vi "Laser_COM.vi"() -> ()   [LabVIEW 2014]
uses:
  <vilib>/Instr/_visa.llb/Select Event Type.ctl
  <vilib>/Instr/_visa.llb/VISA Configure Serial Port (Instr).vi
panel:
  out "7":bool
  out "6":bool
  out "4":bool
  out "5":bool
  out "3":bool
  out "2":bool
  out "1":bool
  out "0":bool
  in  "Control PL":bool
  out "DB25 PL":bool
  out "RS232 PL":bool
  out "DB25 GL":bool
  out "RS232 GL":bool
  in  "Control GL":bool
  out "DB25 ML":bool
  out "RS232 ML":bool
  in  "Control ML":bool
  out "on/off? 5":bool
  in  "Laser":bool
  out "Laser EM":bool caption="Излучение включено!"
  out "on/off? 3":bool
  out "on/off? 2":bool
  in  "Send":bool
  in  "write buffer":string caption="Передать команду"
  out "COM_connect":bool
  in  "Connect":bool
  out "SN:":string
  out "ID:":string
  out "Guide  laser":bool
  out "module temp":dbl caption="Темп. модуля" format="%#_g °C"
  in  "Power":dbl(slide) caption="Мощность излучения, %" min=0.0 max=100.0 step=0.5 scale=0.0..100.0 scale format="%#.2g"
  in  "Laser pilot":bool caption="Лазер пилот"
  in  "COM":refnum<visa-resource-name>="COM1" caption="Laser COM-port"
  out "read buffer":string caption="ОТВЕТ:"
  out "error out":errorcluster
  in  "error in (no error)":errorcluster
  # "ID:\n\nSN:"
  # "Блок  управления основным лазером"
  # "RS-232"
  # "DB-25"
  # "T модуля -"
  # "RS-232"
  # "Мощьность  излучения, %"
  # "DB-25"
  # "DB-25"
  # "Пилот Лазер"
  # "RS-232"
  # "DB-25"
  # "Терминал"
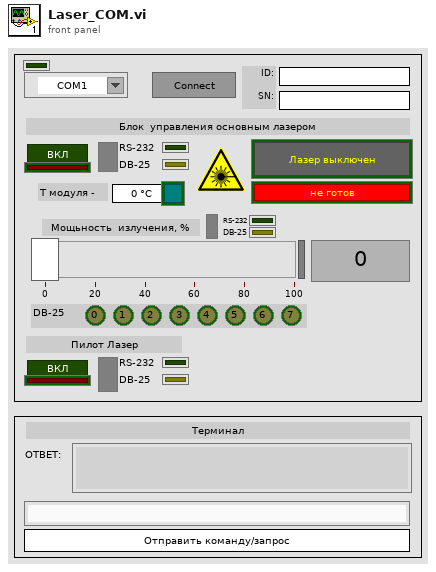
[diagram p1: front panel]
types:
  T1 = typedef "Select Event Type.ctl" = u32
  T2 = cluster{"Power control by DB-25":bool, "Reserved[1]":bool, "AuxOFF control by DB-25":bool, "Guide laser control by DB-25":bool, "Reserved[4]":bool, "Reserved[5]":bool, "Reserved[6]":bool, "Emission Modulation control by DB-25":bool, "The laser is in Jump PRR mode":bool, "Reserved[9]":bool, "Bitstream 1 (BS1) mode is active":bool, "Reserved[11]":bool, "PRR controlled by Sync line in DB-25":bool, "Emission Enable control by DB-25":bool, "APD mode is controlled by DB-25":bool, "Automatic latch":bool, "Reserved[16]":bool, "Reserved[17]":bool, "Reserved[18]":bool, "The laser is in Sweep PRR mode":bool, "The laser is in Follow PRR mode":bool, "Manual Prepump mode is active":bool, "Manual residual is controlled by DB-25":bool, "Reserved[23]":bool, "Reserved[24]":bool, "Guide laser safety function is not activated":bool, "Discharge circuit safety function is activated":bool, "Reserved[27]":bool, "Reserved[28]":bool, "Reserved[29]":bool, "Reserved[30]":bool, "Reserved[31]":bool}
  T3 = cluster{"Rack  reflection":bool, "Temp Laser module":bool, "Temp Laser head":bool, "System Alarm":bool, "+24V main supply Alarm":bool, "HK supply  Alarm":bool, "Laser ready":bool, "Warning is activated":bool}
  T4 = cluster{"Emergency stop":bool, "External PRR [1]":bool, "External PRR [2]":bool, "Reserved [3]":bool, "Reserved [4]":bool, "Guide laser":bool, "Reserved [6]":bool, "Reserved [7]":bool, "Laser emission":bool, "Reserved [9]":bool, "Reserved [10]":bool, "Laser emission command was received by RS-232":bool, "Guide laser command was received by RS-232":bool, "24V Main supply voltage is in specified range":bool, "HK supply voltage is in specified range":bool, "Emission Enable is switched by RS-232":bool, "Reserved [16]":bool, "Reserved [17]":bool, "Reserved [18]":bool, "Reserved [19]":bool, "Reserved [20]":bool, "Reserved [21]":bool, "Reserved [22]":bool, "Reserved [23]":bool, "Reserved [24]":bool, "Reserved [25]":bool, "Reserved [26]":bool, "Reserved [27]":bool, "Reserved [28]":bool, "Reserved [29]":bool, "Reserved [30]":bool, "Reserved [31]":bool}
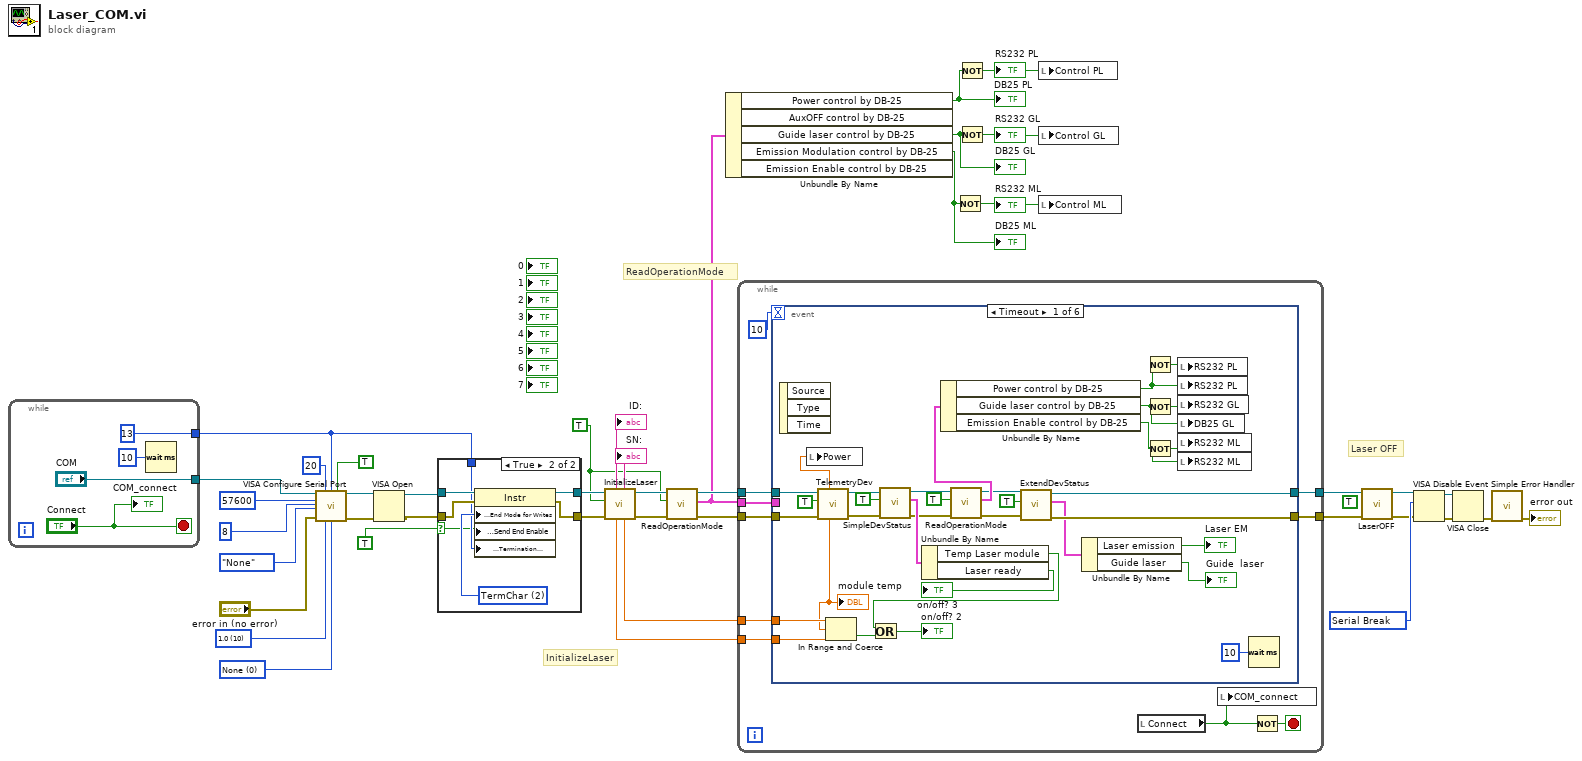
[diagram p0: block diagram]
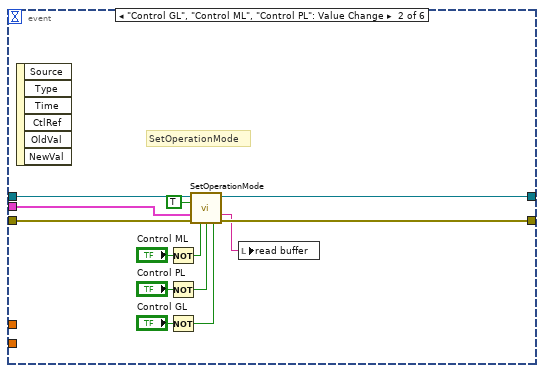
[diagram p2: hidden frame]
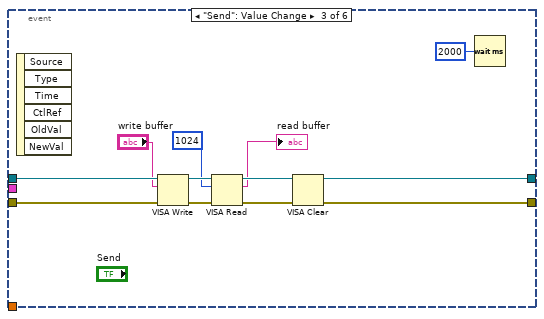
[diagram p3: hidden frame]
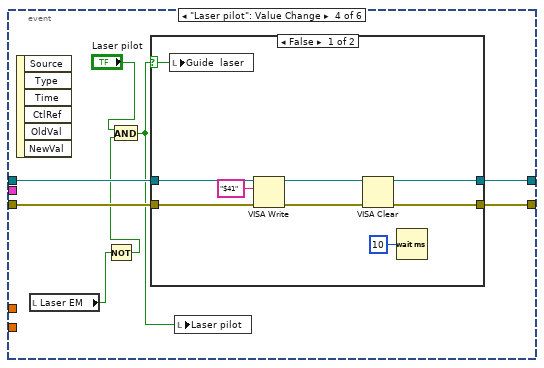
[diagram p4: hidden frame]
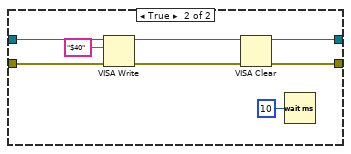
[diagram p5: hidden frame]
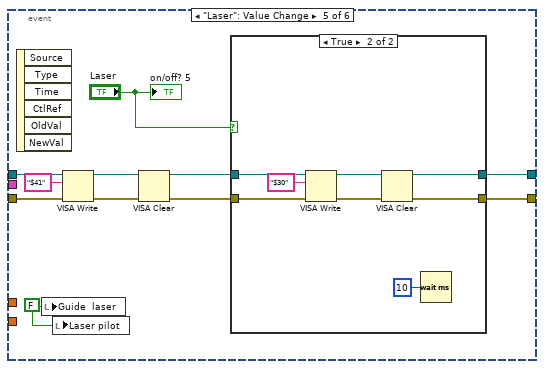
[diagram p6: hidden frame]
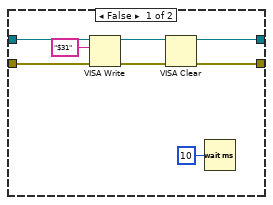
[diagram p7: hidden frame]
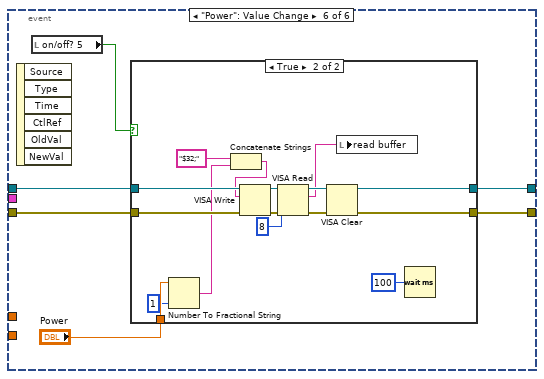
[diagram p8: hidden frame]
diagram:
  w23 = T1 1073684515 items=["Service Request"=1073684491, "Trigger"=3221168138, "Clear"=1073684493, "VXI Signal"=1073684512, "VXI/VME Interrupt"=3221168161, "VXI/VME Sysfail"=1073684509, "VXI/VME Sysreset"=1073684510, "GPIB CIC"=1073684498, "GPIB Talk"=1073684499, "GPIB Listen"=1073684500, "PXI Interrupt"=1073684514, "Serial Break"=1073684515, "Serial TermChar"=1073684516, "Serial CTS"=1073684521, "Serial DSR"=1073684522, "Serial DCD"=1073684524, "Serial RI"=1073684526, "Serial Character"=1073684533, "USB Interrupt"=1073684535, "All Enabled"=1073709055] ("Event Type")
  (unwired) TRUE
  w28 = u16 0 items=["None", "XON/XOFF", "RTS/CTS", "XON/XOFF & RTS/CTS", "DTR/DSR", "XON/XOFF & DTR/DSR"] ("flow control (0:none)")
  w10 = TRUE
  w35 = u16 10 items=["1.0"=10, "1.5"=15, "2.0"=20] ("stop bits (10: 1 bit)")
  # "Laser OFF"
  # "ReadOperationMode"
  # "InitializeLaser"
  n1 = while {
    tunnel: ["COM"] -> w27
    tunnel: [i16 13 ("term_char")] -> w26
    stop <- "Connect" stop-if-true
    n2 = Wait (ms)(milliseconds to wait=u32 10) -> ()  [unwired: 1 out]
    "COM_connect" <- "Connect"
  }
  n3 = call-poly "VISA Configure Serial Port"("VISA resource name"=w27, "timeout (10sec)"=u32 20, "termination char\n(0xA = '\\n' = LF)"=w26, "Enable Termination\nChar (T)"=TRUE ("Enable Termination\nChar (T)"), "baud rate (9600)"=u32 57600 ("baud rate"), "data bits (8)"=u16 8, "parity (0:none)"=enum16{"None", "Odd", "Even", "Mark", "Space"}."None", "error in (no error)"="error in (no error)", "stop bits (10: 1 bit)"=w35, "flow control (0:none)"=w28) -> ("VISA resource name out"=w38:refnum<visa-resource-name>, "error out"=w37:errorcluster)  [unwired: 4 in]
  n4 = VISA Open(error in (no error)=w37, VISA resource name=w38) -> (VISA resource name=w32:refnum<visa-resource-name>, error out=w33:errorcluster)  [unwired: 3 in]
  n5 = case shown="True" TRUE ("End write with termination character?") {
    selector: TRUE ("End write with termination character?") -> [_ w49]
    tunnel: w32 -> [w47 w55]
    tunnel: w33 -> [w48 w54]
    tunnel: [w47 w53] -> w21
    tunnel: [w48 w52] -> w22
    tunnel: w26 -> [_ w50]
    frame False {
    }
    frame True {
      w51 = u16 2 items=["None", "LastBit", "TermChar", "Break"] ("Serial Settings:Serial End Mode for Writes")
      n6 = property class="Instr"(reference=w55, error in=w54, "Serial Settings:End Mode for Writes"=w51, "Message Based Settings:Send End Enable"=w49, "Message Based Settings:Termination Character"=w50) -> (reference out=w53:refnum<visa-resource-name>, error out=w52:errorcluster)
    }
  }
  n7 = call "InitializeLaser.vi"("error in"=w22, "ON/OFF"=w10, "VISA resource name in"=w21) -> ("error out"=w11:errorcluster, "VISA resource name out"=w12:refnum<visa-resource-name>, "Tmax"=w20:dbl, "SN:"=→"SN:":string, "Tmin"=w19:dbl, "Лазер: ID:"=→"ID:":string)  [unwired: 1 in, 2 out]
  n8 = call "ReadOperationMode.vi"("error in"=w11, "ON/OFF"=w10, "VISA resource name in"=w12) -> ("error out"=w13:errorcluster, "Operation Mode Status"=w3:T2, "VISA resource name out"=w14:refnum<visa-resource-name>)  [unwired: 5 in, 1 out]
  n9 = Unbundle By Name(w3) -> ("Power control by DB-25"=w9:bool, "Guide laser control by DB-25"=w7:bool, "Emission Modulation control by DB-25"=w4:bool)  [unwired: 2 out]
  "DB25 GL" <- w7
  "DB25 PL" <- w9
  "DB25 ML" <- w4
  n10 = while {
    tunnel: w13 -> [w60]
    tunnel: w14 -> [w61]
    tunnel: [w63] -> w16
    tunnel: [w62] -> w15
    tunnel: w20 -> [w58]
    tunnel: w19 -> [w57]
    tunnel: w3 -> [w56]
    stop <- w65 stop-if-true
    n11 = event shown="[0] Timeout" {
      selector: _ -> [_ _ _ _ _ _]
      dyn-events: _ -> [_ _ _ _ _ _]
      timeout: 10 -> [_ _ _ _ _ _]
      tunnel: w61 -> [w74 w112 w124 w132 w159 w181]
      tunnel: w60 -> [w73 w111 w123 w131 w158 w180]
      tunnel: [w78 w109 w118 w130 w154 w179] -> w63
      tunnel: [w77 w110 w117 w129 w153 w178] -> w62
      tunnel: w57 -> [w97 _ _ _ _ _]
      tunnel: w58 -> [w98 _ _ _ _ _]
      tunnel: w56 -> [_ w106 _ _ _ _]
      event Timeout {
        n12 = event-data() -> ()  [unwired: 1 in, 3 out]
        n13 = call "TelemetryDev.vi"("error in"=w73, "ON/OFF"=TRUE, "VISA resource name in"=w74) -> ("error out"=w70:errorcluster, "VISA resource name out"=w71:refnum<visa-resource-name>, "module temp"=w69:dbl, "Laser Power,%"=w68:dbl)  [unwired: 4 in, 1 out]
        "module temp" <- w69
        n14 = local write "Power"(w68) -> ()
        n15 = In Range and Coerce(upper limit=w98, x=w69, lower limit=w97) -> (In Range?=w81:bool)  [unwired: 1 out]
        n16 = call "SimpleDevStatus.vi"("error in"=w70, "ON/OFF"=TRUE ("Boolean"), "VISA resource name in"=w71) -> ("error out"=w90:errorcluster, "Device Status"=w93:T3, "VISA resource name out"=w91:refnum<visa-resource-name>)  [unwired: 5 in]
        n17 = Unbundle By Name(w93) -> ("Temp Laser module"=w95:bool, "Laser ready"=→"on/off? 3":bool)
        n18 = Or(x=w95, y=w81) -> (x .or. y?=→"on/off? 2":bool)
        n19 = call "ReadOperationMode.vi"("error in"=w90, "ON/OFF"=TRUE, "VISA resource name in"=w91) -> ("error out"=w79:errorcluster, "Operation Mode Status"=w88:T2, "VISA resource name out"=w80:refnum<visa-resource-name>)  [unwired: 5 in, 1 out]
        n20 = Unbundle By Name(w88) -> ("Power control by DB-25"=w86:bool, "Guide laser control by DB-25"=w84:bool, "Emission Enable control by DB-25"=w82:bool)
        n21 = call "ExtendDevStatus.vi"("error in"=w79, "ON/OFF"=TRUE, "VISA resource name in"=w80) -> ("error out"=w77:errorcluster, "Extend Device Status"=w75:T4, "VISA resource name out"=w78:refnum<visa-resource-name>)  [unwired: 5 in]
        n22 = Unbundle By Name(w75) -> ("Laser emission"=→"Laser EM":bool, "Guide laser"=→"Guide  laser":bool)
        n23 = Not(x=w86) -> (.not. x?=w87:bool)
        n24 = Not(x=w84) -> (.not. x?=w85:bool)
        n25 = Not(x=w82) -> (.not. x?=w83:bool)
        n26 = local write "RS232 PL"(w87) -> ()
        n27 = local write "RS232 PL"(w86) -> ()
        n28 = local write "RS232 GL"(w85) -> ()
        n29 = local write "DB25 GL"(w84) -> ()
        n30 = local write "RS232 ML"(w83) -> ()
        n31 = local write "RS232 ML"(w82) -> ()
        n32 = Wait (ms)(milliseconds to wait=u32 10) -> ()  [unwired: 1 out]
      }
      event "Control GL", "Control ML", "Control PL": Value Change {
        # "SetOperationMode"
        n33 = event-data() -> ()  [unwired: 1 in, 6 out]
        n34 = Not(x="Control ML") -> (.not. x?=w101:bool)
        n35 = Not(x="Control PL") -> (.not. x?=w100:bool)
        n36 = Not(x="Control GL") -> (.not. x?=w104:bool)
        n37 = call "SetOperationMode.vi"("VISA resource name in"=w112, "ON/OFF"=TRUE, "Operation Mode Status"=w106, "error in"=w111, "Laser"=w101, "Power"=w100, "Guide laser"=w104) -> ("VISA resource name out"=w109:refnum<visa-resource-name>, "Message"=w107:string, "error out"=w110:errorcluster)  [unwired: 6 in]
        n38 = local write "read buffer"(w107) -> ()
      }
      event "Send": Value Change {
        n39 = event-data() -> ()  [unwired: 1 in, 6 out]
        n40 = VISA Write(VISA resource name=w124, write buffer="write buffer", error in (no error)=w123) -> (VISA resource name out=w122:refnum<visa-resource-name>, error out=w121:errorcluster)  [unwired: 1 out]
        n41 = VISA Read(VISA resource name=w122, byte count=u32 1024, error in (no error)=w121) -> (VISA resource name out=w120:refnum<visa-resource-name>, read buffer=→"read buffer":string, error out=w119:errorcluster)  [unwired: 1 out]
        n42 = VISA Clear(VISA resource name=w120, error in (no error)=w119) -> (VISA resource name out=w118:refnum<visa-resource-name>, error out=w117:errorcluster)
        n43 = Wait (ms)(milliseconds to wait=u32 2000) -> ()  [unwired: 1 out]
      }
      event "Laser pilot": Value Change {
        n44 = event-data() -> ()  [unwired: 1 in, 6 out]
        n45 = local read "Laser EM"() -> (w128:bool)
        n46 = Not(x=w128) -> (.not. x?=w126:bool)
        n47 = And(x="Laser pilot", y=w126) -> (x .and. y?=w125:bool)
        n48 = case shown="False" w125 {
          selector: w125 -> [w139 _]
          tunnel: w132 -> [w141 w149]
          tunnel: w131 -> [w140 w148]
          tunnel: [w136 w145] -> w130
          tunnel: [w135 w144] -> w129
          frame False {
            n49 = local write "Guide  laser"(w139) -> ()
            n50 = VISA Write(VISA resource name=w141, write buffer="$41", error in (no error)=w140) -> (VISA resource name out=w134:refnum<visa-resource-name>, error out=w133:errorcluster)  [unwired: 1 out]
            n51 = VISA Clear(VISA resource name=w134, error in (no error)=w133) -> (VISA resource name out=w136:refnum<visa-resource-name>, error out=w135:errorcluster)
            n52 = Wait (ms)(milliseconds to wait=u32 10 ("millisecond multiple")) -> ()  [unwired: 1 out]
          }
          frame True {
            n53 = VISA Write(VISA resource name=w149, write buffer="$40", error in (no error)=w148) -> (VISA resource name out=w143:refnum<visa-resource-name>, error out=w142:errorcluster)  [unwired: 1 out]
            n54 = VISA Clear(VISA resource name=w143, error in (no error)=w142) -> (VISA resource name out=w145:refnum<visa-resource-name>, error out=w144:errorcluster)
            n55 = Wait (ms)(milliseconds to wait=u32 10 ("millisecond multiple")) -> ()  [unwired: 1 out]
          }
        }
        n56 = local write "Laser pilot"(w125) -> ()
      }
      event "Laser": Value Change {
        w152 = FALSE ("on/off?")
        n57 = event-data() -> ()  [unwired: 1 in, 6 out]
        n58 = local write "Guide  laser"(w152) -> ()
        n59 = local write "Laser pilot"(w152) -> ()
        n60 = VISA Write(VISA resource name=w159, write buffer="$41", error in (no error)=w158) -> (VISA resource name out=w151:refnum<visa-resource-name>, error out=w150:errorcluster)  [unwired: 1 out]
        n61 = VISA Clear(VISA resource name=w151, error in (no error)=w150) -> (VISA resource name out=w156:refnum<visa-resource-name>, error out=w155:errorcluster)
        n62 = case shown="True" "Laser" {
          tunnel: w156 -> [w167 w175]
          tunnel: w155 -> [w166 w174]
          tunnel: [w165 w173] -> w154
          tunnel: [w164 w172] -> w153
          frame False {
            n63 = VISA Write(VISA resource name=w167, write buffer="$31", error in (no error)=w166) -> (VISA resource name out=w161:refnum<visa-resource-name>, error out=w162:errorcluster)  [unwired: 1 out]
            n64 = VISA Clear(VISA resource name=w161, error in (no error)=w162) -> (VISA resource name out=w165:refnum<visa-resource-name>, error out=w164:errorcluster)
            n65 = Wait (ms)(milliseconds to wait=u32 10) -> ()  [unwired: 1 out]
          }
          frame True {
            n66 = VISA Write(VISA resource name=w175, write buffer="$30", error in (no error)=w174) -> (VISA resource name out=w170:refnum<visa-resource-name>, error out=w169:errorcluster)  [unwired: 1 out]
            n67 = VISA Clear(VISA resource name=w170, error in (no error)=w169) -> (VISA resource name out=w173:refnum<visa-resource-name>, error out=w172:errorcluster)
            n68 = Wait (ms)(milliseconds to wait=u32 10) -> ()  [unwired: 1 out]
          }
        }
        "on/off? 5" <- "Laser"
      }
      event "Power": Value Change {
        n69 = event-data() -> ()  [unwired: 1 in, 6 out]
        n70 = local read "on/off? 5"() -> (w182:bool)
        n71 = case shown="True" w182 {
          tunnel: w181 -> [w184 w196]
          tunnel: w180 -> [w183 w195]
          tunnel: [w184 w194] -> w179
          tunnel: [w183 w193] -> w178
          tunnel: "Power" -> [_ w190]
          frame False {
          }
          frame True {
            n72 = Number To Fractional String(number=w190, precision (6)=i16 1) -> (F-format string=w189:string)  [unwired: 2 in]
            n73 = Concatenate Strings("$32;" ("write buffer"), w189) -> (w191:string)
            n74 = VISA Write(VISA resource name=w196, write buffer=w191, error in (no error)=w195) -> (VISA resource name out=w198:refnum<visa-resource-name>, error out=w197:errorcluster)  [unwired: 1 out]
            n75 = VISA Read(VISA resource name=w198, byte count=u32 8, error in (no error)=w197) -> (VISA resource name out=w199:refnum<visa-resource-name>, read buffer=w186:string, error out=w200:errorcluster)  [unwired: 1 out]
            n76 = VISA Clear(VISA resource name=w199, error in (no error)=w200) -> (VISA resource name out=w194:refnum<visa-resource-name>, error out=w193:errorcluster)
            n77 = local write "read buffer"(w186) -> ()
            n78 = Wait (ms)(milliseconds to wait=u32 100) -> ()  [unwired: 1 out]
          }
        }
      }
    }
    n79 = local read "Connect"() -> (w64:bool)
    n80 = local write "COM_connect"(w64) -> ()
    n81 = Not(x=w64) -> (.not. x?=w65:bool)
  }
  n82 = Not(x=w4) -> (.not. x?=w5:bool)
  "RS232 ML" <- w5
  n83 = Not(x=w9) -> (.not. x?=w8:bool)
  "RS232 PL" <- w8
  n84 = Not(x=w7) -> (.not. x?=w6:bool)
  "RS232 GL" <- w6
  n85 = local write "Control PL"(w8) -> ()
  n86 = local write "Control GL"(w6) -> ()
  n87 = local write "Control ML"(w5) -> ()
  n88 = call "LaserOFF.vi"("error in"=w15, "VISA resource name in"=w16) -> ("error out"=w1:errorcluster, "VISA resource name out"=w2:refnum<visa-resource-name>)  [unwired: 8 in]
  n89 = VISA Disable Event(8:w1, 10:w23, 11:w2) -> (0:w24:errorcluster, 3:w25:refnum<visa-resource-name>)  [unwired: 1 out]
  n90 = VISA Close(VISA resource name=w25, error in (no error)=w24) -> (error out=w29:errorcluster)
  n91 = call <vilib>:"Simple Error Handler.vi"("error in (no error)"=w29) -> ("error out"=→"error out":errorcluster)  [unwired: 4 in, 4 out]
